vi "Register For Event.vi"(8 "Error In":errorcluster, 9 "Event Name":string, 10 "Registrant Enq":refnum<class "Message Enqueuer.lvclass">, 11 "Event Source Actor In":refnum<class "Event Source Actor.lvclass">) -> (0 "Error Out":errorcluster, 3 "Event Source Actor Out":refnum<class "Event Source Actor.lvclass">)   [LabVIEW 2020, in "Event Source.lvlib" / "Event Source Actor.lvclass"]
doc: "This method registers a specific Actors Enqueuer and a Zero Coupling based message (inheriting from Event Generated Msg.lvclass) to used when the specified Event is Fired anywhere inside the Event Source Actor."
uses:
  Event Source Actor.lvclass
  <vilib>/ActorFramework/Message Enqueuer/Message Enqueuer.lvclass
  Event Source Actor.lvclass/Event Source Actor.ctl
  73deaf50-2c1c-4897-b2f9-f93b2ed11082.vi
  <resource>/AFDebug/AF Debug.lvlib
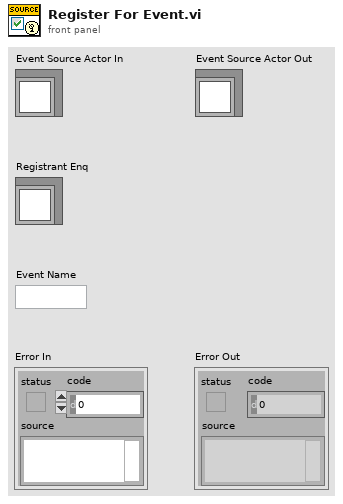
[diagram p1: front panel]
types:
  T1 = map{string, set{refnum<class "Message Enqueuer.lvclass">}}
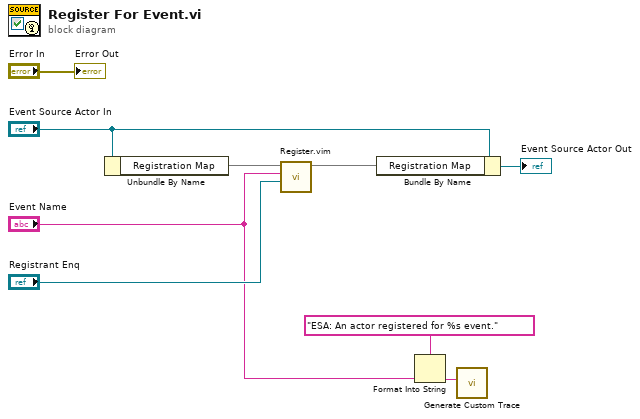
[diagram p0: block diagram]
diagram:
  n1 = Unbundle By Name("Event Source Actor In") -> ("Registration Map"=w6:T1)
  n2 = call "Register.vim"("set element"="Registrant Enq", "key"="Event Name", "map in"=w6) -> ("map out"=w5:T1)  [unwired: 6 in, 2 out]
  n3 = Bundle By Name(cluster="Event Source Actor In", "Registration Map"=w5) -> (→"Event Source Actor Out":refnum<class "Event Source Actor.lvclass">)
  n4 = Format Into String(format string="ESA: An actor registered for %s event." ("Custom Action"), "Event Name") -> (resulting string=w3:string)  [unwired: 2 in, 1 out]
  n5 = call <resource>:"Generate Custom Trace.vi"("Custom Action"=w3) -> ()  [unwired: 11 in]
  "Error Out" <- "Error In"
